vi "ConvertWindowToDisplayWindowCommand.vi"(11 "Window":u8=1 min=1 max=2 step=1) -> (3 "Display Window Command":string)   [LabVIEW 2012, in "Keithley-6482.lvlib"]
uses:
  Keithley-6482.lvlib
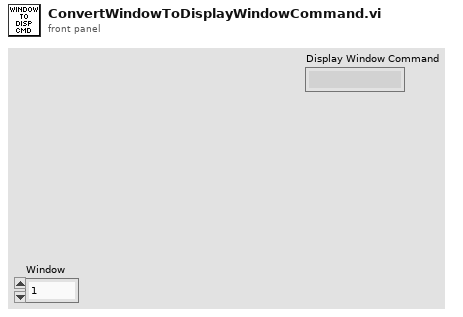
[diagram p1: front panel]
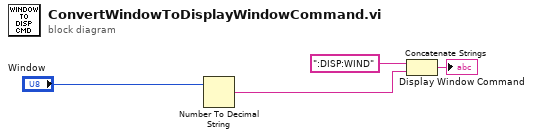
[diagram p0: block diagram]
diagram:
  n1 = Number To Decimal String(number="Window") -> (decimal integer string=w2:string)  [unwired: 1 in]
  n2 = Concatenate Strings(":DISP:WIND", w2) -> (→"Display Window Command":string)
